vi "merge.vi"(8 "error in (no error)":errorcluster, 10 "update":refnum<class "GenericImagingMode.lvclass">, 11 "ImagingModeDL090130Frame in":refnum<class "ImagingModeDL090130Frame.lvclass">=refnum) -> (0 "error out":errorcluster, 3 "ImagingModeDL090130Frame out":refnum<class "ImagingModeDL090130Frame.lvclass">)   [LabVIEW 2010, in "ImagingModeDL090130Frame.lvclass"]
uses:
  ImagingModeDL090130Frame.lvclass
  GenericImagingMode/GenericImagingMode/GenericImagingMode.lvclass
  ImagingModeDL090923Scaffold/ImagingModeDL090923Scaffold/ImagingModeDL090923Scaffold.lvclass
  ImagingModeDL090130Frame.lvclass/ImagingModeDL090130Frame.ctl
  common/classes/ErrorController/ErrorController/class_data.vi
  common/classes/ErrorController/ErrorController/ErrorController.lvclass
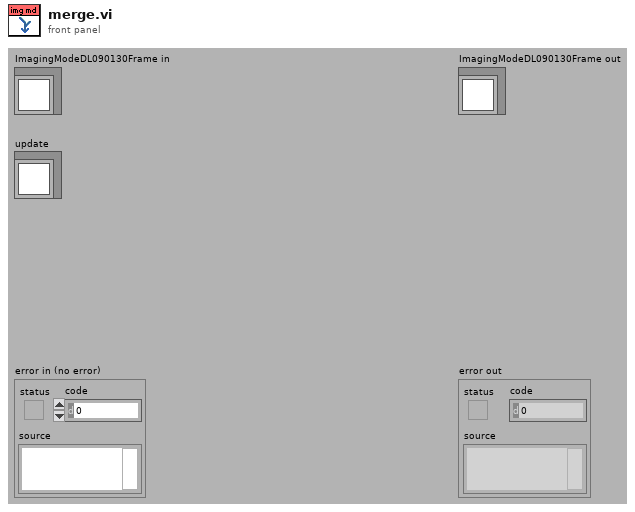
[diagram p1: front panel]
types:
  T1 = typedef "ImagingModeDL090130Frame.lvclass/settings_cluster.ctl" = cluster{"FrameSettings":cluster{"ResolutionX":i32, "ResolutionY":i32, "AspectRatioX":dbl, "AspectRatioY":dbl, "FrameScanRate":dbl[unit]}, "StackSettings":cluster{"Frames":i32, "AveragingRepetitions":i32, "StepSize":dbl[unit], "ReturnToOrigin":bool, "translation mode":T2, "depth/intensity points":cluster{"depth":dbl[unit], "intensity":dbl}[]}}
  T2 = typedef "ImagingModeDL090130Frame.lvclass/translation_mode_enum.ctl" = enum16{"scanHead", "stage"}
  T3 = cluster{"line-scan time":dbl[unit], "pixel-dwell time":dbl[unit]}
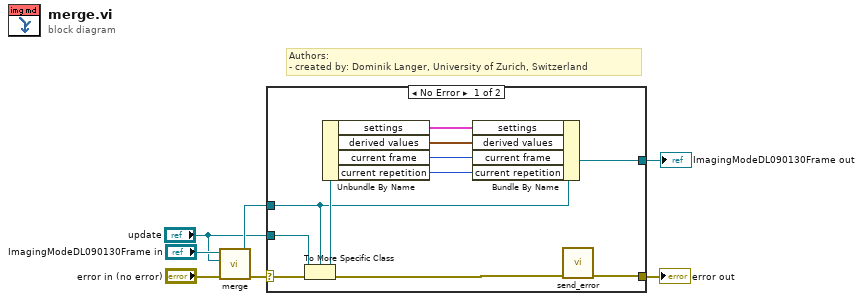
[diagram p0: block diagram]
diagram:
  # "Authors: \n- created by: Dominik Langer, University of Zurich, Switzerland"
  n1 = call-parent "merge.vi"("error in (no error)"="error in (no error)", "update"="update", "GenericScanMode in"="ImagingModeDL090130Frame in") -> ("error out"=w4:errorcluster, "GenericScanMode out"=w2:refnum<class "ImagingModeDL090130Frame.lvclass">)  [unwired: 7 out]
  n2 = case shown="No Error" w4 {
    selector: w4 -> [w17 w20]
    tunnel: [w9 w20] -> w7
    tunnel: [w15 w19] -> w6
    tunnel: w2 -> [w11 w19]
    tunnel: "update" -> [w18 _]
    frame No Error {
      n3 = To More Specific Class(target class=w11, reference=w18, error in=w17) -> (specific class reference=w16:refnum<class "ImagingModeDL090130Frame.lvclass">, error out=w10:errorcluster)
      n4 = Unbundle By Name(w16) -> ("settings"=w14:T1, "derived values"=w8:T3, "current frame"=w13:i32, "current repetition"=w12:i32)
      n5 = Bundle By Name(cluster=w11, "settings"=w14, "derived values"=w8, "current frame"=w13, "current repetition"=w12) -> (w15:refnum<class "ImagingModeDL090130Frame.lvclass">)
      n6 = call "send_error.vi"("error in (no error)"=w10) -> ("error out"=w9:errorcluster)  [unwired: 10 in]
    }
    frame Error {
    }
  }
  "error out" <- w7
  "ImagingModeDL090130Frame out" <- w6
